vi "CellInfoForDrawing.vi"(8 "error in (no error)":errorcluster, 11 "SnakeBodyCell in":refnum<class "SnakeBodyCell.lvclass">) -> (0 "error out":errorcluster, 1 "Position":T1, 2 "Color":u32, 3 "SnakeBodyCell out":refnum<class "SnakeBodyCell.lvclass">)   [LabVIEW 2018, in "SnakeBodyCell.lvclass"]
uses:
  SnakeBodyCell.lvclass
  Typedefs/XYposition.ctl
  SnakeBodyCell.lvclass/SnakeBodyCell.ctl
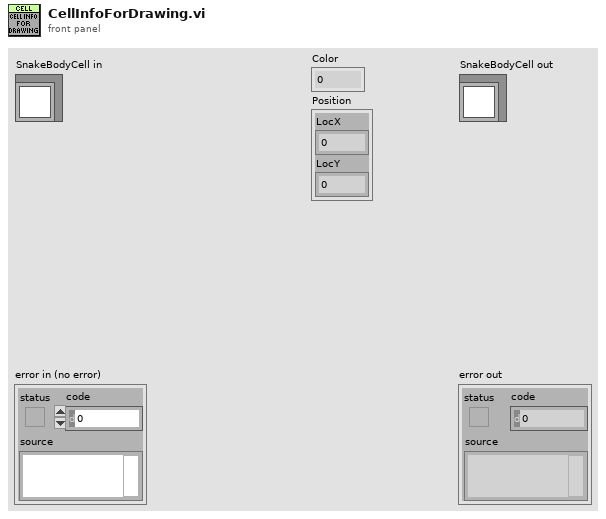
[diagram p1: front panel]
types:
  T1 = typedef "XYposition.ctl" = cluster{"LocX":u16, "LocY":u16}
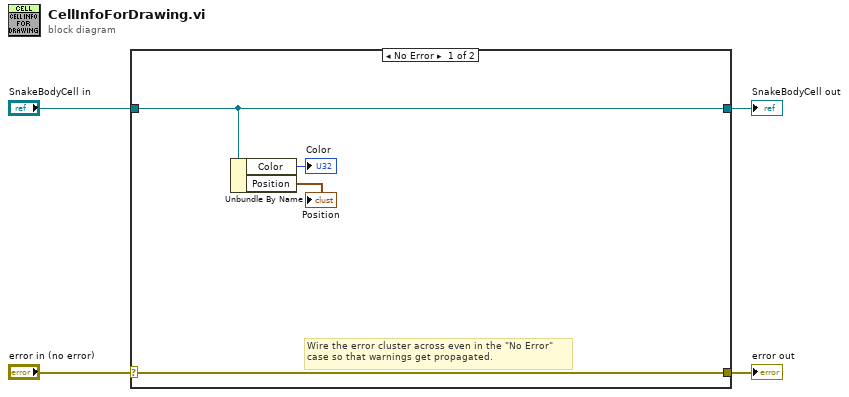
[diagram p0: block diagram]
diagram:
  n1 = case shown="No Error" "error in (no error)" {
    selector: "error in (no error)" -> [w8 w10]
    tunnel: [w8 w10] -> w3
    tunnel: [w7 w9] -> w1
    tunnel: "SnakeBodyCell in" -> [w7 w9]
    frame No Error {
      # "Wire the error cluster across even in the \"No Error\"\ncase so that warnings get propagated."
      n2 = Unbundle By Name(w7) -> ("Color"=→"Color":u32, "Position"=→"Position":T1)
    }
    frame Error {
    }
  }
  "error out" <- w3
  "SnakeBodyCell out" <- w1
